vi "outputCurrent.vi"(8 "error in (no error)":errorcluster, 9 "calibratedValue":dbl, 10 "channel":i32, 11 "K2602 in":refnum<class "K2602.lvclass">) -> (0 "error out":errorcluster, 3 "K2602 out":refnum<class "K2602.lvclass">)   [LabVIEW 2011, in "Hardware.lvlib" / "Channels.lvlib" / "K2602.lvclass"]
uses:
  K2602.lvclass
  K2602.lvclass/K2602.ctl
  <instrlib>/Keithley 2600 Series/Keithley 2600 Series.lvlib
  AnalogOutput.lvclass
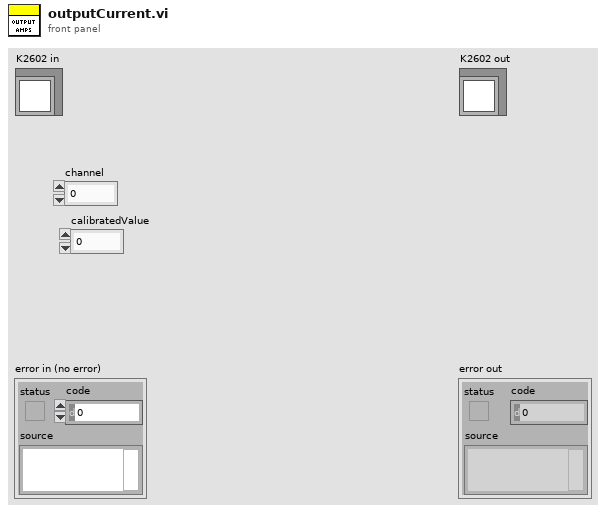
[diagram p1: front panel]
types:
  T1 = cluster{"VoltageLimit":dbl, "CurrentLimit":dbl}[]
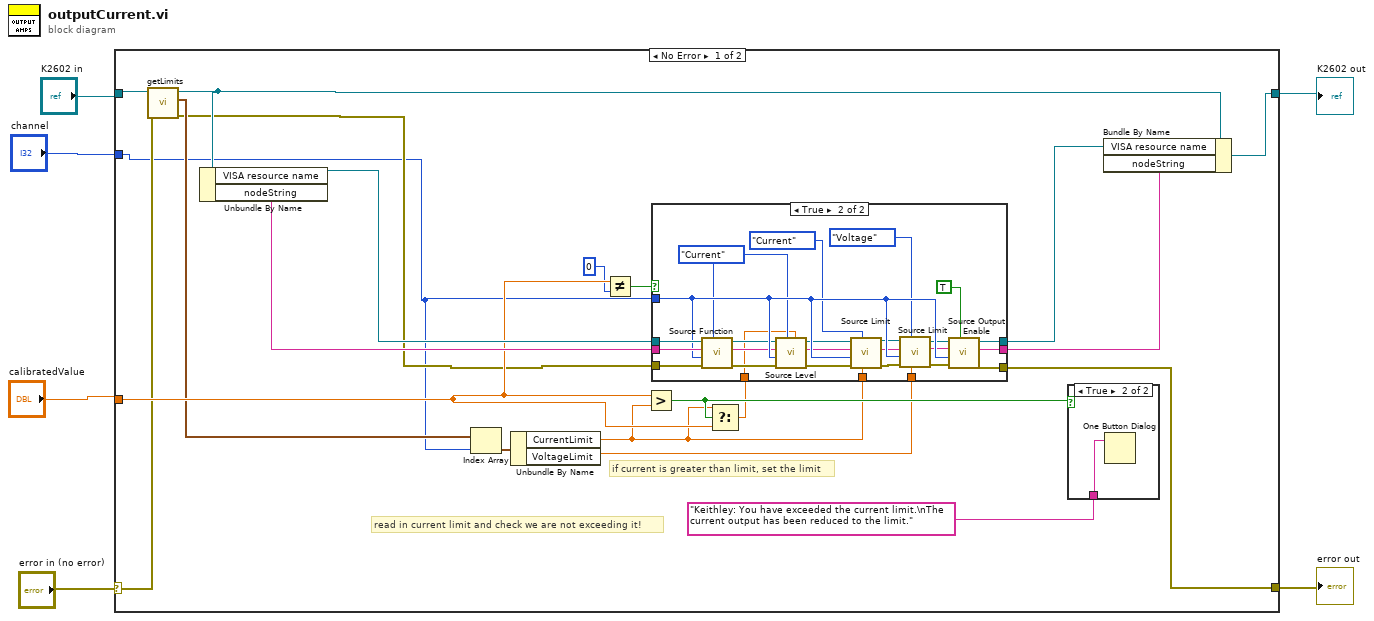
[diagram p0: block diagram]
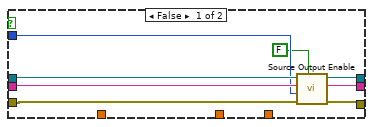
[diagram p2: hidden frame]
diagram:
  n1 = case shown="No Error" "error in (no error)" {
    selector: "error in (no error)" -> [w19 w63]
    tunnel: [w23 w64] -> w3
    tunnel: "K2602 in" -> [w20 w64]
    tunnel: [w22 w63] -> w4
    tunnel: "calibratedValue" -> [w21 _]
    tunnel: "channel" -> [w13 _]
    frame No Error {
      # "if current is greater than limit, set the limit"
      # "read in current limit and check we are not exceeding it!"
      n2 = call "getLimits.vi"("error in (no error)"=w19, "AnalogOutput in"=w20) -> ("error out"=w14:errorcluster, "Limits"=w18:T1, "AnalogOutput out"=w15:refnum<class "K2602.lvclass">)  [unwired: 7 in]
      n3 = Unbundle By Name(w15) -> ("VISA resource name"=w27:refnum<visa-resource-name>, "nodeString"=w26:string)
      n4 = Index Array(array=w18, index=w13) -> (element=w12:cluster{"VoltageLimit":dbl, "CurrentLimit":dbl})
      n5 = Unbundle By Name(w12) -> ("CurrentLimit"=w9:dbl, "VoltageLimit"=w11:dbl)
      n6 = Not Equal?(x=w21, y=0) -> (x != y?=w8:bool)
      n7 = Greater?(x=w21, y=w9) -> (0:w17:bool)
      n8 = Select(t=w9, s=w17, f=w21) -> (s? t:f=w10:dbl)
      n9 = case shown="True" w8 {
        tunnel: w27 -> [w35 w61]
        tunnel: w26 -> [w34 w60]
        tunnel: w14 -> [w33 w59]
        tunnel: [w28 w58] -> w22
        tunnel: [w29 w57] -> w24
        tunnel: [w30 w56] -> w25
        tunnel: w13 -> [w32 w55]
        tunnel: w11 -> [_ w54]
        tunnel: w10 -> [_ w37]
        tunnel: w9 -> [_ w36]
        frame False {
          n10 = call <instrlib>:"Source Output Enable.vi"("Output (Off)"=FALSE, "error in (no error)"=w33, "Channel (Channel A)"=w32, "Node In"=w34, "VISA resource name"=w35) -> ("error out"=w28:errorcluster, "Node Out"=w29:string, "VISA resource name out"=w30:refnum<visa-resource-name>)  [unwired: 3 in, 1 out]
        }
        frame True {
          w48 = enum32{"Current", "Voltage"}."Current" ("Source Function (Current)")
          n11 = call <instrlib>:"Source Function.vi"("Function (Current)"=w48, "error in (no error)"=w59, "Channel (Channel A)"=w55, "Node In"=w60, "VISA resource name"=w61) -> ("error out"=w51:errorcluster, "Node Out"=w53:string, "VISA resource name out"=w52:refnum<visa-resource-name>)  [unwired: 4 out]
          n12 = call <instrlib>:"Source Level.vi"("Level (0.000)"=w37, "Function (Current)"=w48, "error in (no error)"=w51, "Channel (Channel A)"=w55, "Node In"=w53, "VISA resource name"=w52) -> ("error out"=w46:errorcluster, "Node Out"=w49:string, "VISA resource name out"=w50:refnum<visa-resource-name>)  [unwired: 3 out]
          n13 = call <instrlib>:"Source Limit.vi"("Limit (0.000)"=w36, "Function (Current)"=enum32{"Current", "Voltage"}."Current" ("x"), "error in (no error)"=w46, "Channel (Channel A)"=w55, "Node In"=w49, "VISA resource name"=w50) -> ("error out"=w42:errorcluster, "Node Out"=w43:string, "VISA resource name out"=w44:refnum<visa-resource-name>)  [unwired: 3 out]
          n14 = call <instrlib>:"Source Limit.vi"("Limit (0.000)"=w54, "Function (Current)"=enum32{"Current", "Voltage"}."Voltage" ("x"), "error in (no error)"=w42, "Channel (Channel A)"=w55, "Node In"=w43, "VISA resource name"=w44) -> ("error out"=w41:errorcluster, "Node Out"=w39:string, "VISA resource name out"=w40:refnum<visa-resource-name>)  [unwired: 3 out]
          n15 = call <instrlib>:"Source Output Enable.vi"("Output (Off)"=TRUE, "error in (no error)"=w41, "Channel (Channel A)"=w55, "Node In"=w39, "VISA resource name"=w40) -> ("error out"=w58:errorcluster, "Node Out"=w57:string, "VISA resource name out"=w56:refnum<visa-resource-name>)  [unwired: 3 in, 1 out]
        }
      }
      n16 = case shown="True" w17 {
        tunnel: "Keithley: You have exceeded the current limit.\nThe current output has been reduced to the limit." -> [_ w62]
        frame False {
        }
        frame True {
          n17 = One Button Dialog(message=w62) -> ()  [unwired: 1 in, 1 out]
        }
      }
      n18 = Bundle By Name(cluster=w15, "VISA resource name"=w25, "nodeString"=w24) -> (w23:refnum<class "K2602.lvclass">)
    }
    frame Error {
    }
  }
  "error out" <- w4
  "K2602 out" <- w3
